vi "taplo.vi"() -> ()   [LabVIEW 2018]
uses:
  Control 2.ctl
  C:/Users/tuan9/Downloads/LabviewHONDA/LabviewHONDA/speedrpmthoLABVIEW/turnright.ctl
  Control 1.ctl
  Control 4.ctl
  Control 3.ctl
  <vilib>/Instr/_visa.llb/VISA Configure Serial Port (Instr).vi
panel:
  out "Numeric 2":dbl
  out "speed 2":dbl
  out "Numeric":dbl
  out "rpm":dbl
  out "gas pendal 4":T1 scale=0.0..100.0
  out "load 3":T2
  out "rpm 2":T3 caption="Gauge" scale=0.0..8.0
  in  "VISA resource name":refnum<visa-resource-name>
  in  "stop":bool
  out "Boolean 4":bool
  out "Right 4":T4
  out "LEFT 4":bool
  out "speed":T5 scale=0.0..180.0
  # "%"
  # "%"
  # "Gas Pendal"
  # "Load"
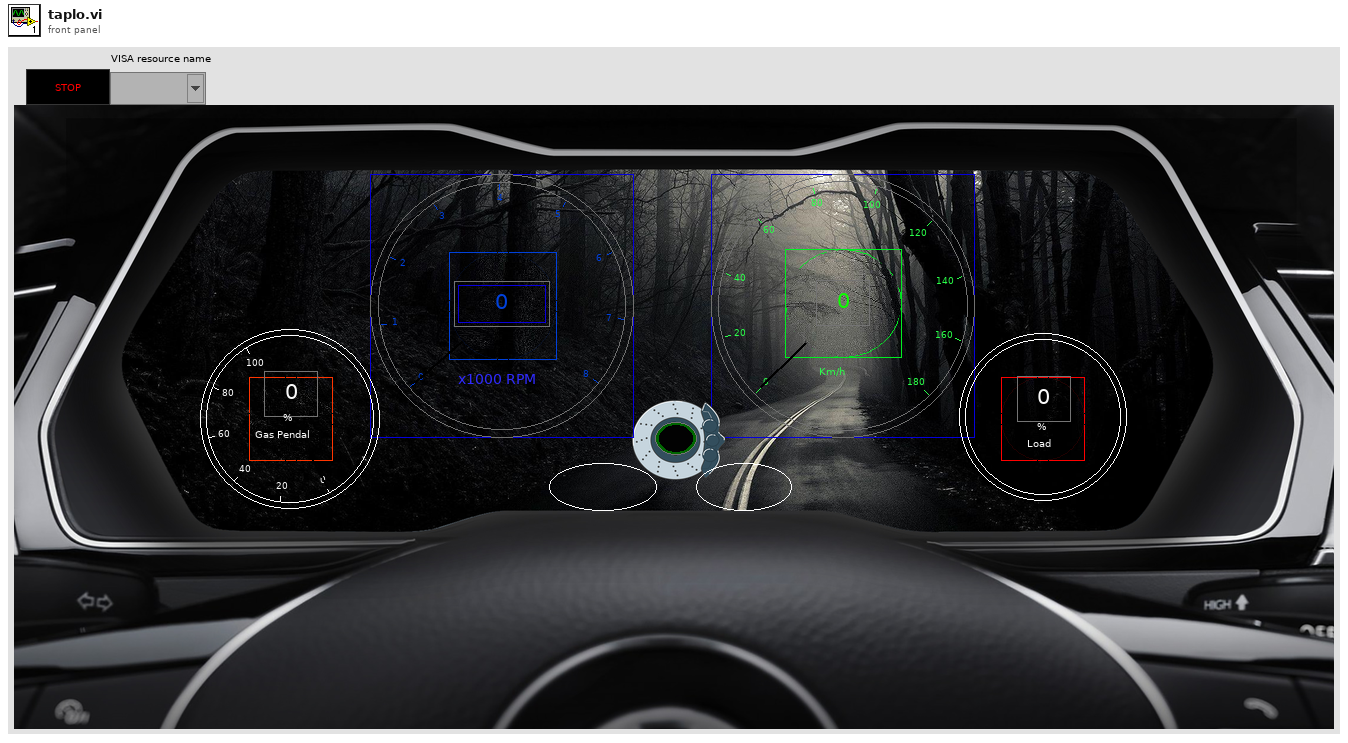
[diagram p1: front panel]
types:
  T1 = typedef "Control 3.ctl" = dbl
  T2 = typedef "Control 4.ctl" = dbl
  T3 = typedef "Control 1.ctl" = dbl
  T4 = typedef "turnright.ctl" = bool
  T5 = typedef "Control 2.ctl" = dbl
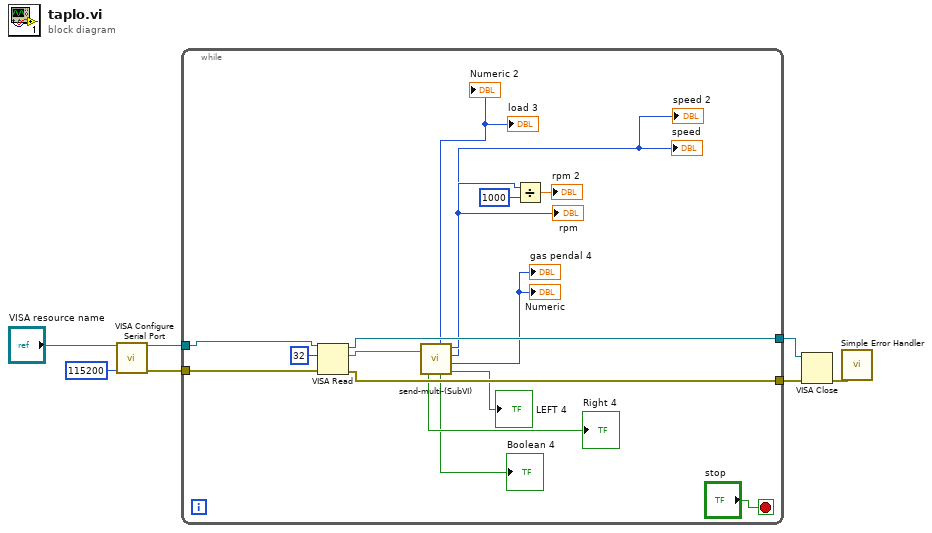
[diagram p0: block diagram]
diagram:
  n1 = call-poly "VISA Configure Serial Port"("VISA resource name"="VISA resource name", "baud rate (9600)"=u32 115200) -> ("VISA resource name out"=w7:refnum<visa-resource-name>, "error out"=w6:errorcluster)  [unwired: 12 in]
  n2 = while {
    tunnel: w7 -> [w22]
    tunnel: w6 -> [w21]
    tunnel: [w18] -> w5
    tunnel: [w17] -> w4
    stop <- "stop" stop-if-true
    n3 = VISA Read(VISA resource name=w22, byte count=u32 32, error in (no error)=w21) -> (VISA resource name out=w18:refnum<visa-resource-name>, read buffer=w20:string, error out=w17:errorcluster)  [unwired: 1 out]
    n4 = call "send-multi-(SubVI).vi"("read buffer"=w20) -> ("Boolean 2"=→"Right 4":bool, "Numeric 4"=→"load 3" →"Numeric 2":i32, "Boolean"=→"Boolean 4":bool, "Numeric 2"=w11:i32, "Numeric 3"=→"speed" →"speed 2":i32, "Numeric"=→"gas pendal 4" →"Numeric":i32, "Boolean 3"=→"LEFT 4":bool)
    "rpm" <- w11
    n5 = Divide(x=w11, y=1000) -> (x/y=→"rpm 2":dbl)
  }
  n6 = VISA Close(VISA resource name=w5, error in (no error)=w4) -> (error out=w1:errorcluster)
  n7 = call <vilib>:"Simple Error Handler.vi"("error in (no error)"=w1) -> ()  [unwired: 4 in, 5 out]
